vi "Write.vi"(8 "error in (no error)":errorcluster, 9 "Value":u16, 10 "ILC in":refnum<class "ILC.lvclass">, 11 "ILC DAC 3 in":refnum<class "ILC DAC 3.lvclass">) -> (0 "error out":errorcluster, 2 "ILC out":refnum<class "ILC.lvclass">, 3 "ILC DAC 3 out":refnum<class "ILC DAC 3.lvclass">)   [LabVIEW 2015, in "ILC DAC 3.lvclass"]
uses:
  ILC DAC 3.lvclass
  <userlib>/Common/ILC/ILC/ILC.lvclass
  <userlib>/Common/ILC/ILC/ILC.lvclass/ILC.ctl
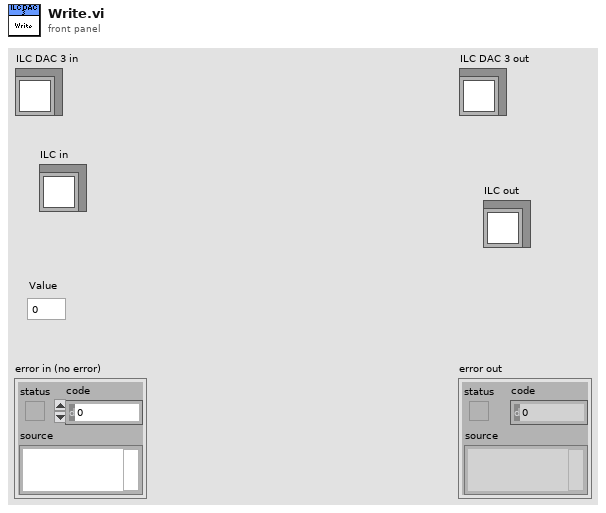
[diagram p1: front panel]
types:
  T1 = typedef "ILCCommon.lvlib/ILCTypedefs.lvlib/Outputs.ctl" = cluster{"Step & Direction":i16, "Blower RPM":u8, "PWM (SSR)":u8, "Ch1":u16, "Ch2":u16, "Ch3":u16, "Ch4":u16}
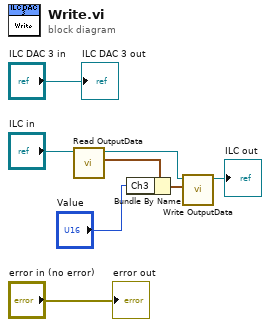
[diagram p0: block diagram]
diagram:
  n1 = call <userlib>:"Read OutputData.vi"("ILC in"="ILC in") -> ("OutputData"=w7:T1, "ILC out"=w8:refnum<class "ILC.lvclass">)  [unwired: 9 in]
  n2 = Bundle By Name(cluster=w7, "Ch3"="Value") -> (w6:T1)
  n3 = call <userlib>:"Write OutputData.vi"("OutputData"=w6, "ILC in"=w8) -> ("ILC out"=→"ILC out":refnum<class "ILC.lvclass">)  [unwired: 9 in]
  "error out" <- "error in (no error)"
  "ILC DAC 3 out" <- "ILC DAC 3 in"
